vi "Inactivity Timer FGV.vi"(10 "Time Target (s)":dbl=10.0 format="%#_13g", 11 "Reset":bool) -> (2 "Time has Elapsed":bool, 3 "Elapsed Time (s)":dbl)   [LabVIEW 2025]
doc: "Inactivity FGV to be used to auto exit from ATM session."
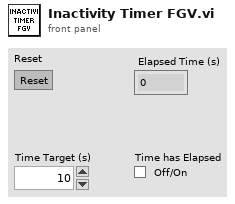
[diagram p1: front panel]
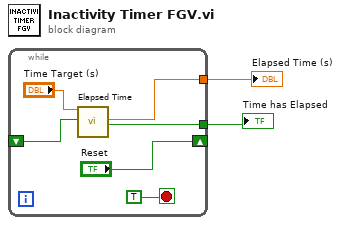
[diagram p0: block diagram]
diagram:
  n1 = while {
    shift-right: ["Reset"] -> _
    shift-left: _ -> [w5]
    tunnel: [w4] -> w2
    tunnel: [w3] -> w1
    stop <- TRUE stop-if-true
    n2 = call "Elapsed Time"("Time Target (s)"="Time Target (s)", "Reset"=w5) -> ("Elapsed Time (s)"=w4:dbl, "Time has Elapsed"=w3:bool)  [unwired: 10 in, 6 out]
  }
  "Elapsed Time (s)" <- w2
  "Time has Elapsed" <- w1
